vi "CS4_BField_Readout.vi"(4 "error in":errorcluster, 7 "GPIB Address":i16) -> (0 "B field read":dbl, 1 "B field read":string, 2 "Set B":dbl, 3 "Set B":string, 5 "error out":errorcluster)   [LabVIEW 2012]
uses:
  Oxford_itc503/BUSGEN.LLB/OxfordAddress.ctl
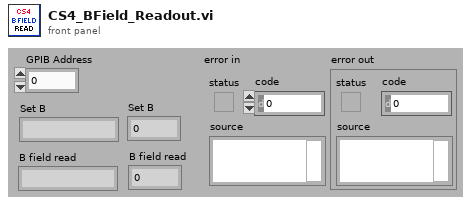
[diagram p1: front panel]
types:
  T1 = typedef "OxfordAddress.ctl" = cluster{"Com Port":i32, "ISOBUS Address":i32, "GPIB Address":i16, "Communication":enum16{"RS232", "ISOBUS", "GPIB", "Gateway"}}
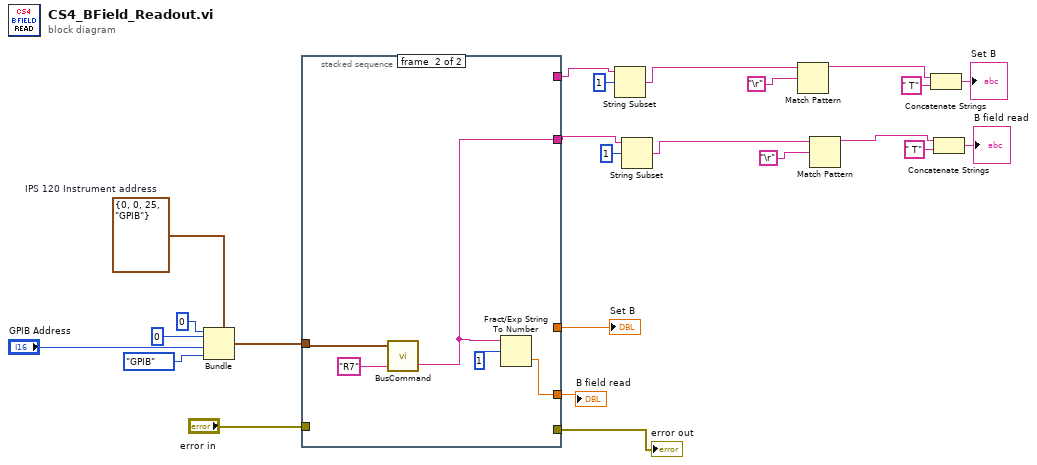
[diagram p0: block diagram]
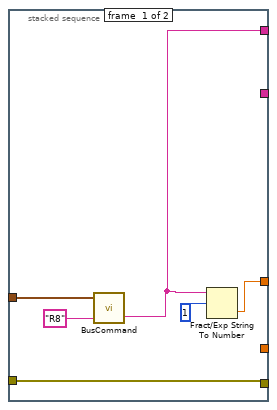
[diagram p2: hidden frame]
diagram:
  w11 = T1 {"Com Port"=0, "ISOBUS Address"=0, "GPIB Address"=25, "Communication"=enum."GPIB"}  # IPS 120 Instrument address
  n1 = Bundle(cluster=w11, "Com Port"=0, "ISOBUS Address"=0, "GPIB Address"="GPIB Address", "Communication"=enum16{"RS232", "ISOBUS", "GPIB", "Gateway"}."GPIB") -> (w20:T1)
  n2 = stacked-sequence {
    tunnel: w20 -> [w27 w33]
    tunnel: "error in" -> [w30 _]
    tunnel: [w30 _] -> w18
    tunnel: [w26 _] -> w4
    tunnel: [_ w32] -> w3
    tunnel: [w25 _] -> w15
    tunnel: [_ w31] -> w14
    frame #0 {
      n3 = call "BusCommand.vi"("Command"="R8", "Instrument address (in)"=w27) -> ("Reply"=w26:string)  [unwired: 1 out]
      n4 = Fract/Exp String To Number(string=w26, offset=1) -> (number=w25:dbl)  [unwired: 2 in, 1 out]
    }
    frame #1 {
      n5 = call "BusCommand.vi"("Command"="R7", "Instrument address (in)"=w33) -> ("Reply"=w32:string)  [unwired: 1 out]
      n6 = Fract/Exp String To Number(string=w32, offset=1) -> (number=w31:dbl)  [unwired: 2 in, 1 out]
    }
  }
  "error out" <- w18
  "Set B" <- w15
  "B field read" <- w14
  n7 = String Subset(string=w4, offset (0)=1) -> (substring=w6:string)  [unwired: 1 in]
  n8 = String Subset(string=w3, offset (0)=1) -> (substring=w5:string)  [unwired: 1 in]
  n9 = Match Pattern(string=w6, regular expression="\r") -> (before substring=w2:string)  [unwired: 1 in, 3 out]
  n10 = Match Pattern(string=w5, regular expression="\r") -> (before substring=w1:string)  [unwired: 1 in, 3 out]
  n11 = Concatenate Strings(w2, " T" ("string")) -> (→"Set B":string)
  n12 = Concatenate Strings(w1, " T" ("string")) -> (→"B field read":string)
